vi "Format Numeric.vi"(6 "Variant in":variant, 7 "Shift Pressed?":bool, 8 "error in (no error)":errorcluster, 10 "QD Combo Box Ref":refnum<vi>, 11 "QD Launch VI Ref":refnum<vi>) -> (0 "error out":errorcluster, 4 "Variant out":variant)   [LabVIEW 2014, in "Format Numeric.lvlib"]
doc: "Formats selected numeric controls, indicators, and/or constants selected. The format descriptor must be entered in the Quick Drop window before activating this plugin.\n\nDefault Shortcut - [N]"
uses:
  Format Numeric.lvlib
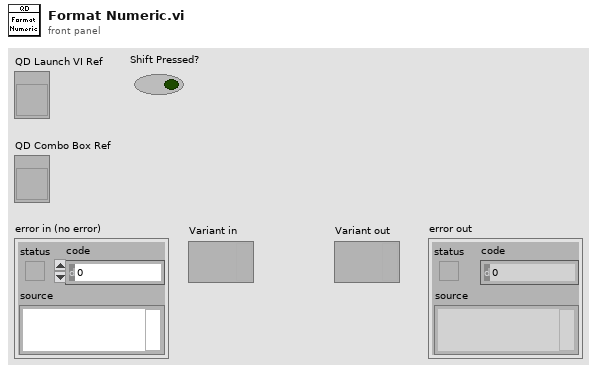
[diagram p1: front panel]
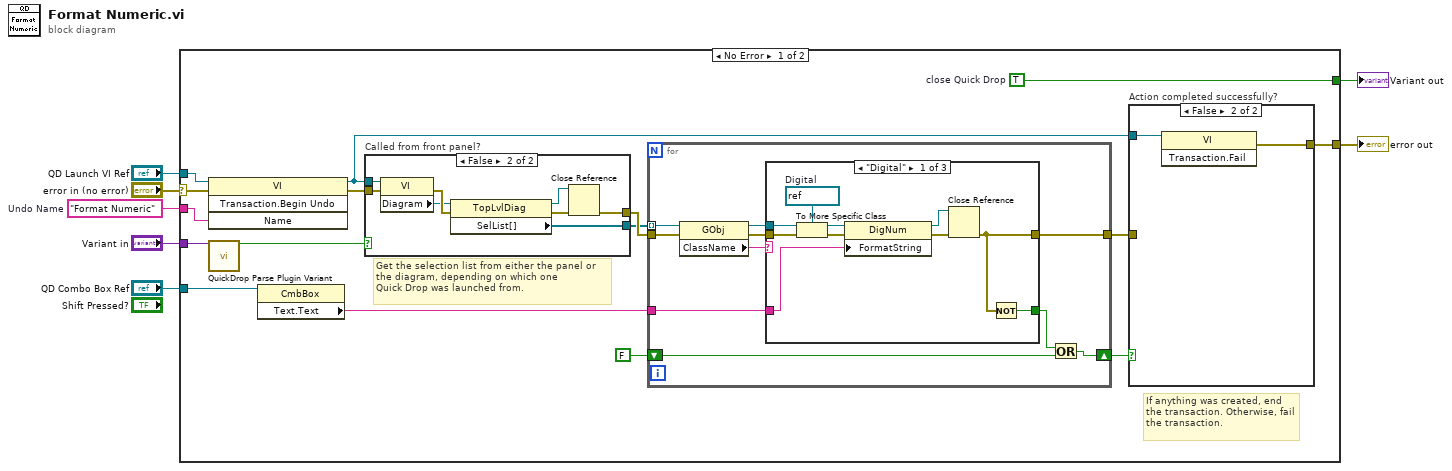
[diagram p0: block diagram]
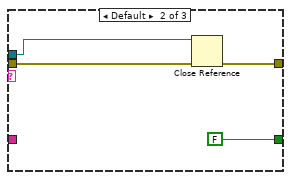
[diagram p2: hidden frame]
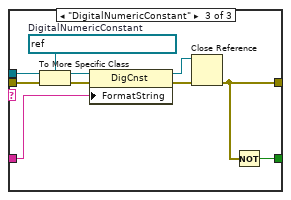
[diagram p3: hidden frame]
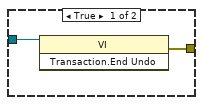
[diagram p4: hidden frame]
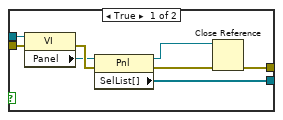
[diagram p5: hidden frame]
diagram:
  w2 = "Format Numeric"  # Undo Name
  n1 = case shown="No Error" "error in (no error)" {
    selector: "error in (no error)" -> [w22 w78]
    tunnel: [w20 w78] -> w6
    tunnel: "QD Launch VI Ref" -> [w17 _]
    tunnel: "QD Combo Box Ref" -> [w9 _]
    tunnel: "Variant in" -> [w23 _]
    tunnel: w2 -> [w16 _]
    tunnel: [w15 _] -> w1
    frame No Error {
      w15 = TRUE  # close Quick Drop
      # "Get the selection list from either the panel or\nthe diagram, depending on which one \nQuick Drop was launched from."
      # "If anything was created, end the transaction. Otherwise, fail the transaction."
      n2 = invoke class="VI" method="Transaction.Begin Undo"(reference=w17, error in=w22, "Name"=w16) -> (reference out=w13:refnum<vi>, error out=w21:errorcluster)  [unwired: 1 in, 2 out]
      n3 = call <vilib>:"QuickDrop Parse Plugin Variant.vi"("QDKS Variant in"=w23) -> ("QD Launch VI Panel?"=w14:bool)  [unwired: 12 in, 2 out]
      n4 = property class="CmbBox"(reference=w9) -> ("Text.Text"=w8:string)  [unwired: 1 in, 2 out]
      n5 = case "Called from front panel?" shown="False" w14 {
        tunnel: w21 -> [w69 w77]
        tunnel: w13 -> [w65 w73]
        tunnel: [w66 w74] -> w19
        tunnel: [w62 w70] -> w10
        frame True {
          n6 = property class="VI"(reference=w65, error in=w69) -> (error out=w68:errorcluster, "Panel"=w64:refnum<vi>)  [unwired: 1 out]
          n7 = property class="Pnl"(reference=w64, error in=w68) -> (reference out=w63:refnum<vi>, error out=w67:errorcluster, "SelList[]"=w62:refnum<vi>[])
          n8 = Close Reference(reference=w63, error in (no error)=w67) -> (error out=w66:errorcluster)
        }
        frame False {
          n9 = property class="VI"(reference=w73, error in=w77) -> (error out=w76:errorcluster, "Diagram"=w72:refnum<vi>)  [unwired: 1 out]
          n10 = property class="TopLvlDiag"(reference=w72, error in=w76) -> (reference out=w71:refnum<vi>, error out=w75:errorcluster, "SelList[]"=w70:refnum<vi>[])
          n11 = Close Reference(reference=w71, error in (no error)=w75) -> (error out=w74:errorcluster)
        }
      }
      n12 = for {
        shift-right: [w29] -> w11
        shift-left: FALSE -> [w30]
        tunnel: w10 -> [w28] mode=indexing
        tunnel: w8 -> [w26]
        tunnel: w19 -> [w33]
        tunnel: [w31] -> w18
        n13 = property class="GObj"(reference=w28, error in=w33) -> (reference out=w27:refnum<vi>, error out=w32:errorcluster, "ClassName"=w24:string)
        n14 = case shown="\"Digital\"" w24 {
          tunnel: w32 -> [w43 w46 w57]
          tunnel: w27 -> [w39 w45 w53]
          tunnel: w26 -> [w36 _ w50]
          tunnel: [w40 w47 w54] -> w31
          tunnel: [w34 FALSE w48] -> w25
          frame "Digital" {
            w37 = refnum<vi> refnum  # Digital
            n15 = To More Specific Class(target class=w37, reference=w39, error in=w43) -> (specific class reference=w38:refnum<vi>, error out=w42:errorcluster)
            n16 = property class="DigNum"(reference=w38, error in=w42, "FormatString"=w36) -> (reference out=w35:refnum<vi>, error out=w41:errorcluster)
            n17 = Close Reference(reference=w35, error in (no error)=w41) -> (error out=w40:errorcluster)
            n18 = Not(x=w40) -> (.not. x?=w34:bool)
          }
          frame Default {
            n19 = Close Reference(reference=w45, error in (no error)=w46) -> (error out=w47:errorcluster)
          }
          frame "DigitalNumericConstant" {
            w51 = refnum<vi> refnum  # DigitalNumericConstant
            n20 = To More Specific Class(target class=w51, reference=w53, error in=w57) -> (specific class reference=w52:refnum<vi>, error out=w56:errorcluster)
            n21 = property class="DigCnst"(reference=w52, error in=w56, "FormatString"=w50) -> (reference out=w49:refnum<vi>, error out=w55:errorcluster)
            n22 = Close Reference(reference=w49, error in (no error)=w55) -> (error out=w54:errorcluster)
            n23 = Not(x=w54) -> (.not. x?=w48:bool)
          }
        }
        n24 = Or(x=w25, y=w30) -> (x .or. y?=w29:bool)
      }
      n25 = case "Action completed successfully?" shown="False" w11 {
        tunnel: w13 -> [w58 w60]
        tunnel: [w59 w61] -> w20
        tunnel: w18 -> [_ _]
        frame True {
          n26 = invoke class="VI" method="Transaction.End Undo"(reference=w58) -> (error out=w59:errorcluster)  [unwired: 2 in, 2 out]
        }
        frame False {
          n27 = invoke class="VI" method="Transaction.Fail"(reference=w60) -> (error out=w61:errorcluster)  [unwired: 2 in, 2 out]
        }
      }
    }
    frame Error {
    }
  }
  "error out" <- w6
  "Variant out" <- w1
